vi "HMI.vi"(8 "error in (no error)":errorcluster caption="entrée d'erreur (pas d'erreur)", 11 "Class Popup Operator_Validation (Default) en entrée":refnum<class "Class Popup Operator_Validation.lvclass">) -> (0 "error out":errorcluster caption="sortie d'erreur", 1 "Input":string, 2 "Operator_Selection":bool, 3 "Class Popup Operator_Validation (Default) en sortie":refnum<class "Class Popup Operator_Validation.lvclass">)   [LabVIEW 2020, in "Library Instrument & Equipement.lvlib" / "Library Popup.lvlib" / "Class Popup Operator_Validation.lvclass"]
uses:
  Class Popup Operator_Validation.lvclass
  C:/Users/ngarcin/OneDrive - Altyor/Standard TB/Class/Popup/Class Popup (Main)/Class Popup (Main).lvclass
  C:/Users/ngarcin/OneDrive - Altyor/Standard TB/Class/Popup/Class Popup Operator_Validation/Class Popup Operator_Validation (Default)/Class Popup Operator_Validation (Virtual).lvclass
  Class Popup Operator_Validation (Default)/Class Popup Operator_Validation (Virtual).lvclass
  Class Popup Operator_Validation.lvclass/Class Popup Operator_Validation.ctl
panel:
  out "Text":string
  out "Image":picture
  in  "Bouton NOK":bool caption="Default"
  in  "Bouton OK":bool caption="Validated"
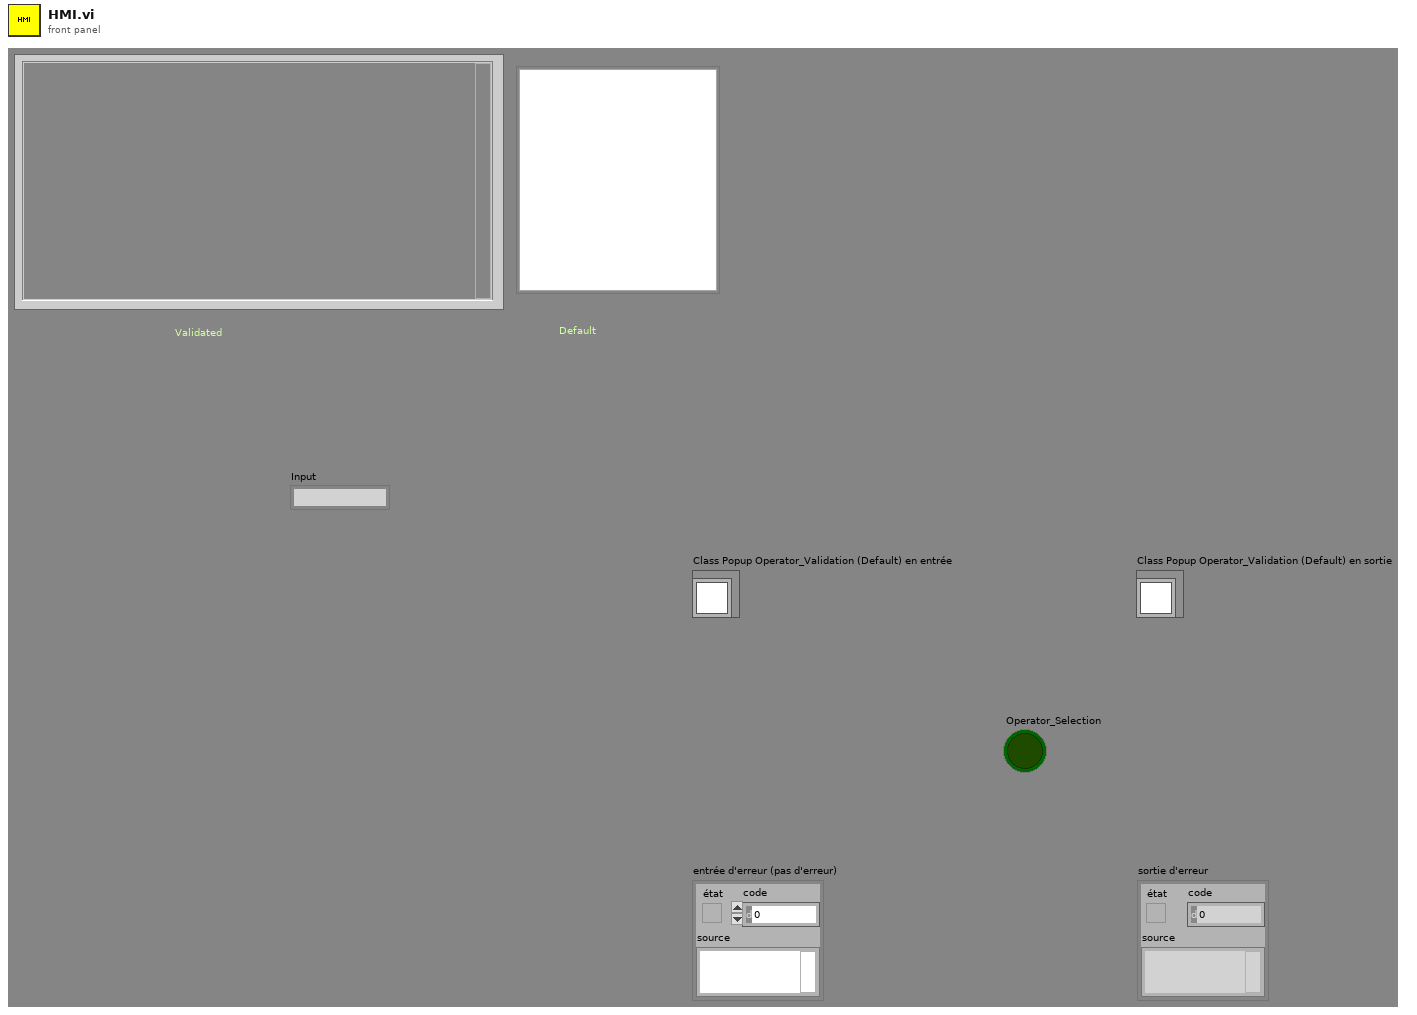
[diagram p1: front panel]
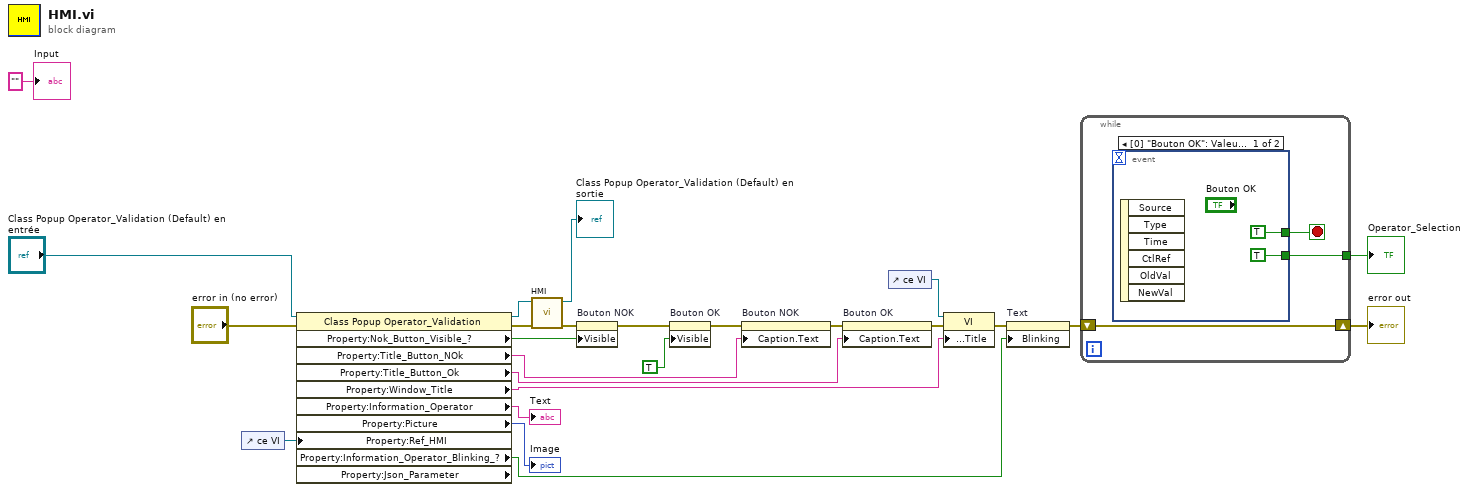
[diagram p0: block diagram]
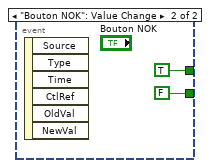
[diagram p2: hidden frame]
diagram:
  n1 = control-ref of="ce VI"() -> (w9:refnum<vi>)
  n2 = property class="Class Popup Operator_Validation" props=["Property:Nok_Button_Visible_?", "Property:Title_Button_NOk", "Property:Title_Button_Ok", "Property:Window_Title", "Property:Information_Operator", "Property:Picture", "Property:Ref_HMI", "Property:Information_Operator_Blinking_?", "Property:Json_Parameter"](reference="Class Popup Operator_Validation (Default) en entrée", error in="error in (no error)", "Property:Ref_HMI"=w9) -> (reference out=w14:refnum<class "Class Popup Operator_Validation.lvclass">, error out=w16:errorcluster, "Property:Nok_Button_Visible_?"=w25:bool, "Property:Title_Button_NOk"=w22:string, "Property:Title_Button_Ok"=w23:string, "Property:Window_Title"=w20:string, "Property:Information_Operator"=→"Text":string, "Property:Picture"=→"Image":picture, "Property:Information_Operator_Blinking_?"=w12:bool)  [unwired: 1 out]
  n3 = call-parent "HMI.vi"("error in (no error)"=w16, "Class Popup Operator_Validation (Default) en entrée"=w14) -> ("error out"=w15:errorcluster, "Class Popup Operator_Validation (Default) en sortie"=→"Class Popup Operator_Validation (Default) en sortie":refnum<class "Class Popup Operator_Validation.lvclass">)  [unwired: 6 in, 2 out]
  n4 = property on="Bouton NOK" class="Bool"(error in=w15, "Visible"=w25) -> (error out=w8:errorcluster)  [unwired: 1 in, 1 out]
  n5 = property on="Bouton OK" class="Bool"(error in=w8, "Visible"=TRUE) -> (error out=w7:errorcluster)  [unwired: 1 in, 1 out]
  n6 = property on="Bouton NOK" class="Bool"(error in=w7, "Caption.Text"=w22) -> (error out=w6:errorcluster)  [unwired: 1 in, 1 out]
  n7 = property on="Bouton OK" class="Bool"(error in=w6, "Caption.Text"=w23) -> (error out=w4:errorcluster)  [unwired: 1 in, 1 out]
  n8 = control-ref of="ce VI"() -> (w5:refnum<vi>)
  n9 = property class="VI"(reference=w5, error in=w4, "Front Panel.Title"=w20) -> (error out=w3:errorcluster)  [unwired: 1 out]
  n10 = property on="Text" class="Ch"(error in=w3, "Blinking"=w12) -> (error out=w2:errorcluster)  [unwired: 1 in, 1 out]
  n11 = while {
    tunnel: [w26] -> w21
    shift-right: [w27] -> w17
    shift-left: w2 -> [w27]
    stop <- w28 stop-if-true
    n12 = event shown="[0] \"Bouton OK\": Valeur changée" {
      selector: _ -> [_ _]
      dyn-events: _ -> [_ _]
      timeout: _ -> [_ _]
      tunnel: [TRUE ("Valeur (Signalisation)") TRUE ("Valeur (Signalisation)")] -> w28
      tunnel: [TRUE ("Operator_Selection") FALSE ("Operator_Selection")] -> w26
      event "Bouton OK": Value Change {
        n13 = event-data() -> ()  [unwired: 1 in, 6 out]
      }
      event "Bouton NOK": Value Change {
        n14 = event-data() -> ()  [unwired: 1 in, 6 out]
      }
    }
  }
  "error out" <- w17
  "Operator_Selection" <- w21
  "Input" <- "" ("Input")
